vi "Set Test Window Topmost.vi"(4 "error in (no error)":errorcluster, 7 "VI Refnum":refnum<vi>) -> (0 "error out":errorcluster, 1 "Window data":T1, 2 "Browser Window":T2, 3 "dup VI Refnum":refnum<vi>)   [LabVIEW 2011]
uses:
  Summitek/Win32/WinUSER/Windows/hWnd.ctl
  Summitek/Win32/WinUSER/Windows/window state.ctl
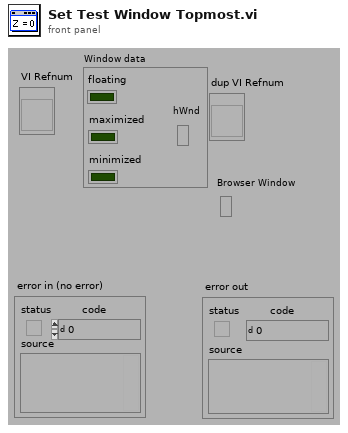
[diagram p1: front panel]
types:
  T1 = typedef "window state.ctl" = cluster{"minimized":bool, "maximized":bool, "floating":bool, "hWnd":T2}
  T2 = typedef "hWnd.ctl" = refnum<k1>
  T3 = enum16{"Get Number of Tasks", "Get Window Info", "Get Window Names"}
  T4 = cluster{"number of windows":i32, "total names length":u32, "number of tasks found":i32, "window handles":u32[], "process ID":u32}
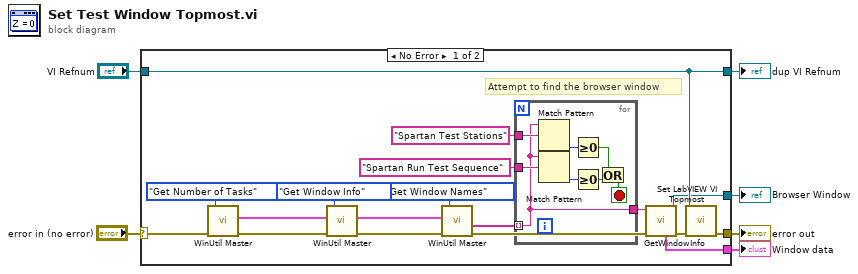
[diagram p0: block diagram]
diagram:
  n1 = case shown="No Error" "error in (no error)" {
    selector: "error in (no error)" -> [w13 w32]
    tunnel: [w23 w33] -> w6
    tunnel: [w7 w32] -> w5
    tunnel: "VI Refnum" -> [w23 w33]
    tunnel: [w9 _] -> w2
    tunnel: [w8 _] -> w1
    frame No Error {
      # "Attempt to find the browser window"
      n2 = call "WinUtil Master.vi"("error in (no error)"=w13, "function"=T3."Get Number of Tasks") -> ("error out"=w17:errorcluster, "window enumeration info out"=w20:T4)  [unwired: 3 in, 1 out]
      n3 = call "WinUtil Master.vi"("error in (no error)"=w17, "window enumeration info in"=w20, "function"=T3."Get Window Info") -> ("error out"=w18:errorcluster, "window enumeration info out"=w19:T4)  [unwired: 2 in, 1 out]
      n4 = call "WinUtil Master.vi"("error in (no error)"=w18, "window enumeration info in"=w19, "function"=T3."Get Window Names") -> ("error out"=w11:errorcluster, "window names"=w12:string[])  [unwired: 2 in, 1 out]
      n5 = for {
        tunnel: "Spartan Run Test Sequence" -> [w31]
        tunnel: "Spartan Test Stations" -> [w30]
        tunnel: w12 -> [w24] mode=indexing
        tunnel: [w24] -> w10
        stop <- w25 stop-if-true
        n6 = Match Pattern(string=w24, regular expression=w30) -> (offset past match=w28:i32)  [unwired: 1 in, 3 out]
        n7 = Match Pattern(string=w24, regular expression=w31) -> (offset past match=w29:i32)  [unwired: 1 in, 3 out]
        n8 = Greater Or Equal To 0?(x=w28) -> (x >= 0?=w27:bool)
        n9 = Greater Or Equal To 0?(x=w29) -> (x >= 0?=w26:bool)
        n10 = Or(x=w27, y=w26) -> (x .or. y?=w25:bool)
      }
      n11 = call "GetWindowInfo.vi"("Window Title (\"\")"=w10) -> ("hWnd"=w8:T2, "Window data"=w9:T1)  [unwired: 6 in, 3 out]
      n12 = call "Set LabVIEW VI Topmost.vi"("error in (no error)"=w11, "VI Refnum (null)"=w23) -> ("error out"=w7:errorcluster)  [unwired: 7 in, 2 out]
    }
    frame Error {
    }
  }
  "error out" <- w5
  "dup VI Refnum" <- w6
  "Browser Window" <- w1
  "Window data" <- w2
